vi "IAI command.vi"(8 "error in (no error)":errorcluster, 10 "packet":string, 11 "VISA Refnum in":refnum<visa-resource-name>) -> (0 "error out":errorcluster, 2 "read buffer":string, 3 "VISA Refnum":refnum<visa-resource-name>)   [LabVIEW 2017]
uses:
  <vilib>/Instr/_visa.llb/VISA Configure Serial Port (Instr).vi
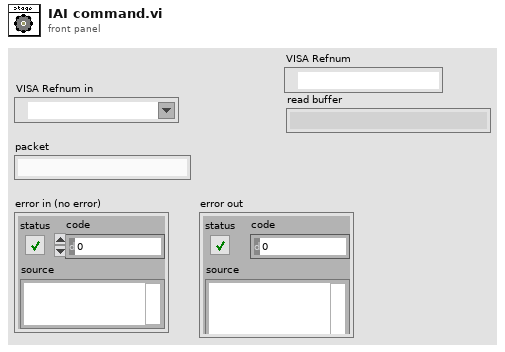
[diagram p1: front panel]
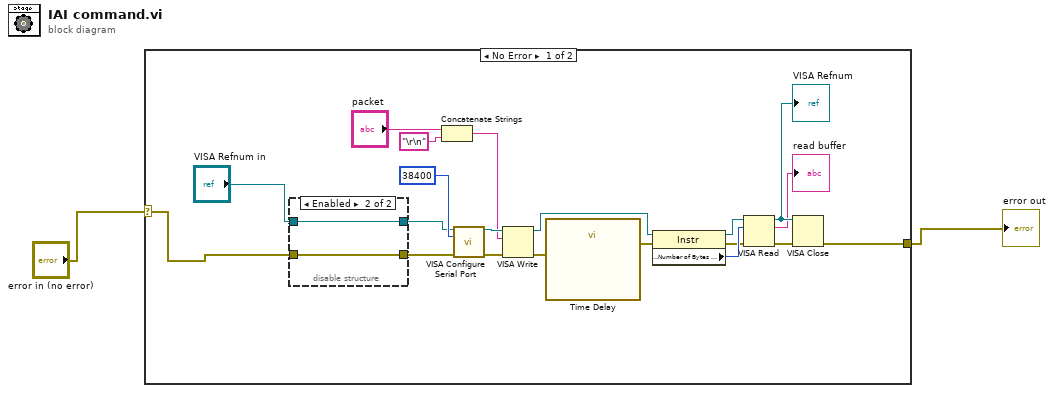
[diagram p0: block diagram]
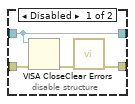
[diagram p2: hidden frame]
diagram:
  n1 = case shown="No Error" "error in (no error)" {
    selector: "error in (no error)" -> [w3 w29]
    tunnel: [w18 w29] -> w2
    frame No Error {
      n2 = disable-structure shown="Enabled" {
        disable-tunnel: w3 -> [w24 w27]
        disable-tunnel: [w25 w27] -> w14
        disable-tunnel: "VISA Refnum in" -> [w23 w28]
        disable-tunnel: [w23 w28] -> w13
        frame Disabled {
          n3 = VISA Close(VISA resource name=w23, error in (no error)=w24) -> (error out=w26:errorcluster)
          n4 = call <vilib>:"Clear Errors.vi"("error in (no error)"=w26) -> ("error out"=w25:errorcluster)  [unwired: 5 in, 1 out]
        }
        frame Enabled {
        }
      }
      n5 = Concatenate Strings("packet", "\r\n" ("string")) -> (w16:string)
      n6 = call-poly "VISA Configure Serial Port"("VISA resource name"=w13, "baud rate (9600)"=u32 38400, "error in (no error)"=w14) -> ("VISA resource name out"=w20:refnum<visa-resource-name>, "error out"=w21:errorcluster)  [unwired: 11 in]
      n7 = VISA Write(VISA resource name=w20, write buffer=w16, error in (no error)=w21) -> (VISA resource name out=w8:refnum<visa-resource-name>, error out=w6:errorcluster)  [unwired: 1 out]
      n8 = call "Time Delay"("error in (no error)"=w6) -> ("error out"=w5:errorcluster)  [unwired: 10 in]
      n9 = property class="Instr"(reference=w8, error in=w5) -> (reference out=w7:refnum<visa-resource-name>, error out=w4:errorcluster, "Serial Settings:Number of Bytes at Serial Port"=w9:u32)
      n10 = VISA Read(VISA resource name=w7, byte count=w9, error in (no error)=w4) -> (VISA resource name out=w11:refnum<visa-resource-name>, read buffer=→"read buffer":string, error out=w22:errorcluster)  [unwired: 1 out]
      "VISA Refnum" <- w11
      n11 = VISA Close(VISA resource name=w11, error in (no error)=w22) -> (error out=w18:errorcluster)
    }
    frame Error {
    }
  }
  "error out" <- w2
